vi "dfd_Classical Filter Design Order Translation.vi"(7 "filter type":T1(ring), 11 "input order":i32=2) -> (3 "order for design":i32)   [LabVIEW 2017, in "NI_DigFilterLicensed.lvlib"]
uses:
  <vilib>/addons/Digital Filter Design/NI_DigFilterLicensed.lvlib
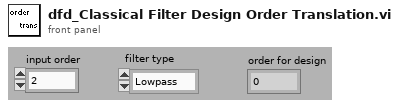
[diagram p1: front panel]
types:
  T1 = enum16{"Lowpass", "Highpass", "Bandpass", "Bandstop"}
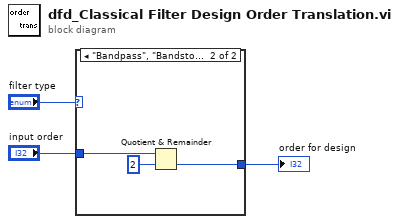
[diagram p0: block diagram]
diagram:
  n1 = case shown="\"Bandpass\", \"Bandstop\"" "filter type" {
    tunnel: "input order" -> [w4 w7]
    tunnel: [w4 w6] -> w1
    frame "Lowpass", "Highpass", Default {
    }
    frame "Bandpass", "Bandstop" {
      n2 = Quotient & Remainder(x=w7, y=2) -> (floor(x/y)=w6:i32)  [unwired: 1 out]
    }
  }
  "order for design" <- w1
